vi "Set AO AI Graph X Axis (WFGraph).vi"(8 "error in (no error)":errorcluster, 10 "X Axis":enum16{"Time", "Samples"}(ring) caption="Enum 3", 11 "WaveformGraph in":refnum<vi>) -> (0 "error out":errorcluster)   [LabVIEW 2019, in "Instrument UI.Lockin.lvclass"]
uses:
  Instrument UI.Lockin.lvclass
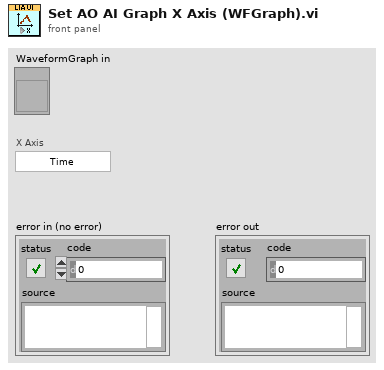
[diagram p1: front panel]
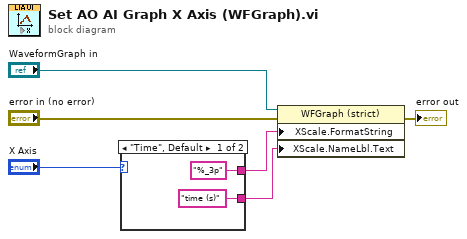
[diagram p0: block diagram]
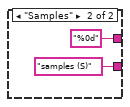
[diagram p2: hidden frame]
diagram:
  n1 = case shown="\"Time\", Default" "X Axis" {
    tunnel: ["%_3p" ("Y Scale.Name Label.Text") "%0d" ("Y Scale.Name Label.Text")] -> w2
    tunnel: ["time (s)" ("Y Scale.Name Label.Text") "samples (S)" ("Y Scale.Name Label.Text")] -> w1
    frame "Time", Default {
    }
    frame "Samples" {
    }
  }
  n2 = property on="Property Node" class="WFGraph (strict)"(reference="WaveformGraph in", error in="error in (no error)", "XScale.FormatString"=w2, "XScale.NameLbl.Text"=w1) -> (error out=→"error out":errorcluster)  [unwired: 1 out]
